vi "Set Sessions VNA.vi"(11 "Semiconductor Module Context":T1) -> (0 "error out":errorcluster, 3 "VNA Instrument Handle Array":refnum<k15>[](array[refnum]))   [LabVIEW 2013]
uses:
  <vilib>/NI_TestStand_SemiconductorModule/NI_TestStand_Semiconductor_Module.lvlibp/PinMap/General/SemiconductorModuleContext.ctl
  Pin Map API/VNA Custom Instrument.lvlib
  <vilib>/NI_TestStand_SemiconductorModule/NI_TestStand_Semiconductor_Module.lvlibp
panel:
  out "Channel Lists":string[](array[string])
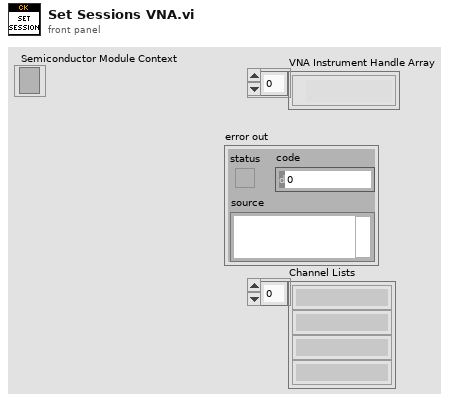
[diagram p1: front panel]
types:
  T1 = typedef "NI_TestStand_Semiconductor_Module.lvlibp/SemiconductorModuleContext.ctl" = refnum<k7>
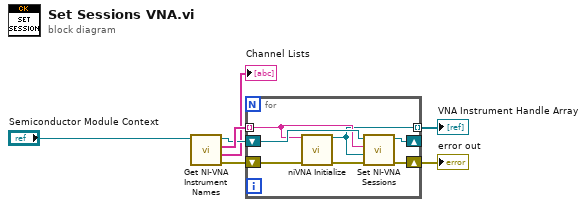
[diagram p0: block diagram]
diagram:
  n1 = call "Get NI-VNA Instrument Names.vi"("Semiconductor Module Context"="Semiconductor Module Context") -> ("error out"=w5:errorcluster, "Channel Lists"=→"Channel Lists":string[], "Instrument Names"=w7:string[], "Semiconductor Module Context Out"=w6:T1)  [unwired: 7 in]
  n2 = for {
    tunnel: w7 -> [w10] mode=indexing
    shift-right: [w9] -> _
    shift-left: w6 -> [w12]
    shift-right: [w11] -> w3
    shift-left: w5 -> [w14]
    tunnel: [w8] -> w2 mode=indexing
    n3 = call <instrlib>:"niVNA Initialize.vi"("resource name"=w10, "error in"=w14) -> ("instrument handle"=w8:refnum<k15>, "error out"=w13:errorcluster)  [unwired: 12 in]
    n4 = call "Set NI-VNA Sessions.vi"("error in (no error)"=w13, "Instrument Session"=w8, "Instrument Name"=w10, "Semiconductor Module Context"=w12) -> ("error out"=w11:errorcluster, "Semiconductor Module Context Out"=w9:T1)  [unwired: 6 in]
  }
  "error out" <- w3
  "VNA Instrument Handle Array" <- w2
